vi "close.vi"(8 "error in (no error)":errorcluster, 11 "FgenNiPxi in":refnum<class "ArbNi.lvclass">) -> (0 "error out":errorcluster)   [LabVIEW 2023, in "ArbNi.lvclass"]
doc: "<b>Author:</b> Wolfgang\n<b>Description:</b> This mimics the abilty to close an instrument reference if opened before."
uses:
  ArbNi.lvclass
  ArbNi.lvclass/ArbNi.ctl
  Arb.lvclass
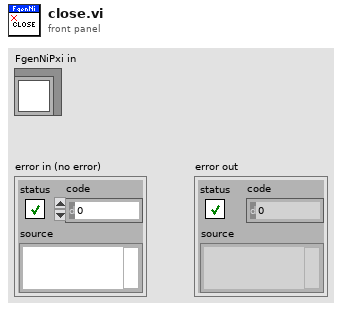
[diagram p1: front panel]
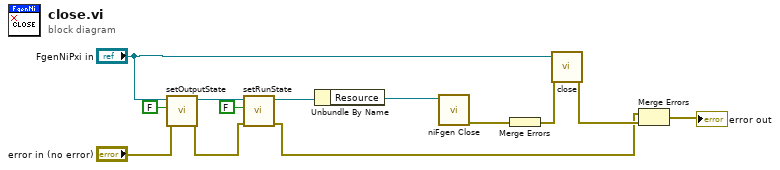
[diagram p0: block diagram]
diagram:
  n1 = call-dynamic "setOutputState.vi"("error in (no error)"="error in (no error)", "Output State"=FALSE, "FgenNiPxi in"="FgenNiPxi in") -> ("error out"=w3:errorcluster, "FgenNiPxi out"=w6:refnum<class "ArbNi.lvclass">)  [unwired: 7 in]
  n2 = call-dynamic "setRunState.vi"("error in (no error)"=w3, "Runstate"=FALSE, "FgenNiPxi in"=w6) -> ("error out"=w2:errorcluster, "FgenNiPxi out"=w5:refnum<class "ArbNi.lvclass">)  [unwired: 7 in]
  n3 = Unbundle By Name(w5) -> ("Resource"=w13:refnum<k15>)
  n4 = call <instrlib>:"niFgen Close.vi"("Instrument Handle"=w13) -> ("error out"=w12:errorcluster)  [unwired: 10 in]
  n5 = Merge Errors(w12) -> (w1:errorcluster)
  n6 = call-parent "close.vi"("error in (no error)"=w1, "Instrument in"="FgenNiPxi in") -> ("error out"=w10:errorcluster)  [unwired: 9 in]
  n7 = Merge Errors(w2, w10) -> (→"error out":errorcluster)
